vi "lab2_sim_modem.vi"() -> ()   [LabVIEW 2014]
uses:
  <vilib>/Addons/Modulation/Digital/General/MT Generate Bits (Galois, PN Order).vi
  <vilib>/Addons/Modulation/Analog/support/mod_Set Error Source.vi
  <vilib>/Addons/Modulation/Digital/Support/Common/Validators/mod_Generate Bits Validate.vi
  <vilib>/Addons/Modulation/Digital/Support/Common/Validators/mod_AWGN Validate.vi
  <vilib>/Addons/Modulation/Digital/Impairments/subVIs/mod_createSeeds.vi
  <vilib>/Addons/Modulation/Digital/Support/Common/Validators/mod_Validate Samples Per Symbol.vi
  <vilib>/Addons/Modulation/Analog/support/Validators/mod_Validate Complex Waveform.vi
  <vilib>/Addons/Modulation/Analog/support/Validators/mod_WFErrorHandler.vi
  <vilib>/Addons/Modulation/Digital/Support/Common/Validators/mod_Generate Filter Coefficients Validate.vi
  <vilib>/Addons/Modulation/Digital/General/subVIs/mod_Generate Filter Coefficients.vi
  <vilib>/Addons/Modulation/Digital/General/subVIs/mod_Generate Bits PN Sequence.vi
  <vilib>/Addons/Modulation/Digital/General/MT Apply Pulse Shaping Filter (Generic).vi
  <vilib>/Analysis/1siggen.llb/Gaussian White Noise (obs 90).vi
  <vilib>/Addons/Modulation/Digital/General/MT Apply Matched Filter (Generic).vi
  <vilib>/addons/Modulation/niDMT.lvlib
panel:
  out "ser/ber":dbl
  out "received symbols":u32
  out "error symbols":i32
  out "ser":dbl
  out "received bits":i32
  out "error bits":i32
  out "ber":dbl format="%#_5e"
  out "sync?":bool
  out "subarray":i16[](array[numeric])
  out "index map":u32[](array[numeric])
  out "output bit stream":i8[](array[numeric])
  in  "modulation":enum16{"PSK", "QAM"}(ring)
  in  "Gray code?":bool=TRUE
  out "size(s)":i32
  out "Received map":cdb[](graph)
  in  "Eb/N0 (10 dB)":dbl=10.0 format="%.2f"
  in  "samples per symbol":i32=16
  in  "filter parameter":dbl=0.5 format="%.2f"
  in  "filter length (symbols)":i32=8
  in  "pulse shaping filter (none)":T1(ring)=enum."Root Raised Cos"
  out "total bits":i32
  in  "total mod symbols":i32=2000 caption="total symbols"
  out "symbol map":cdb[](array[numeric])
  out "Transmitter map":cdb[](graph)
  in  "stop":bool
  in  "M-ARY":i32=4
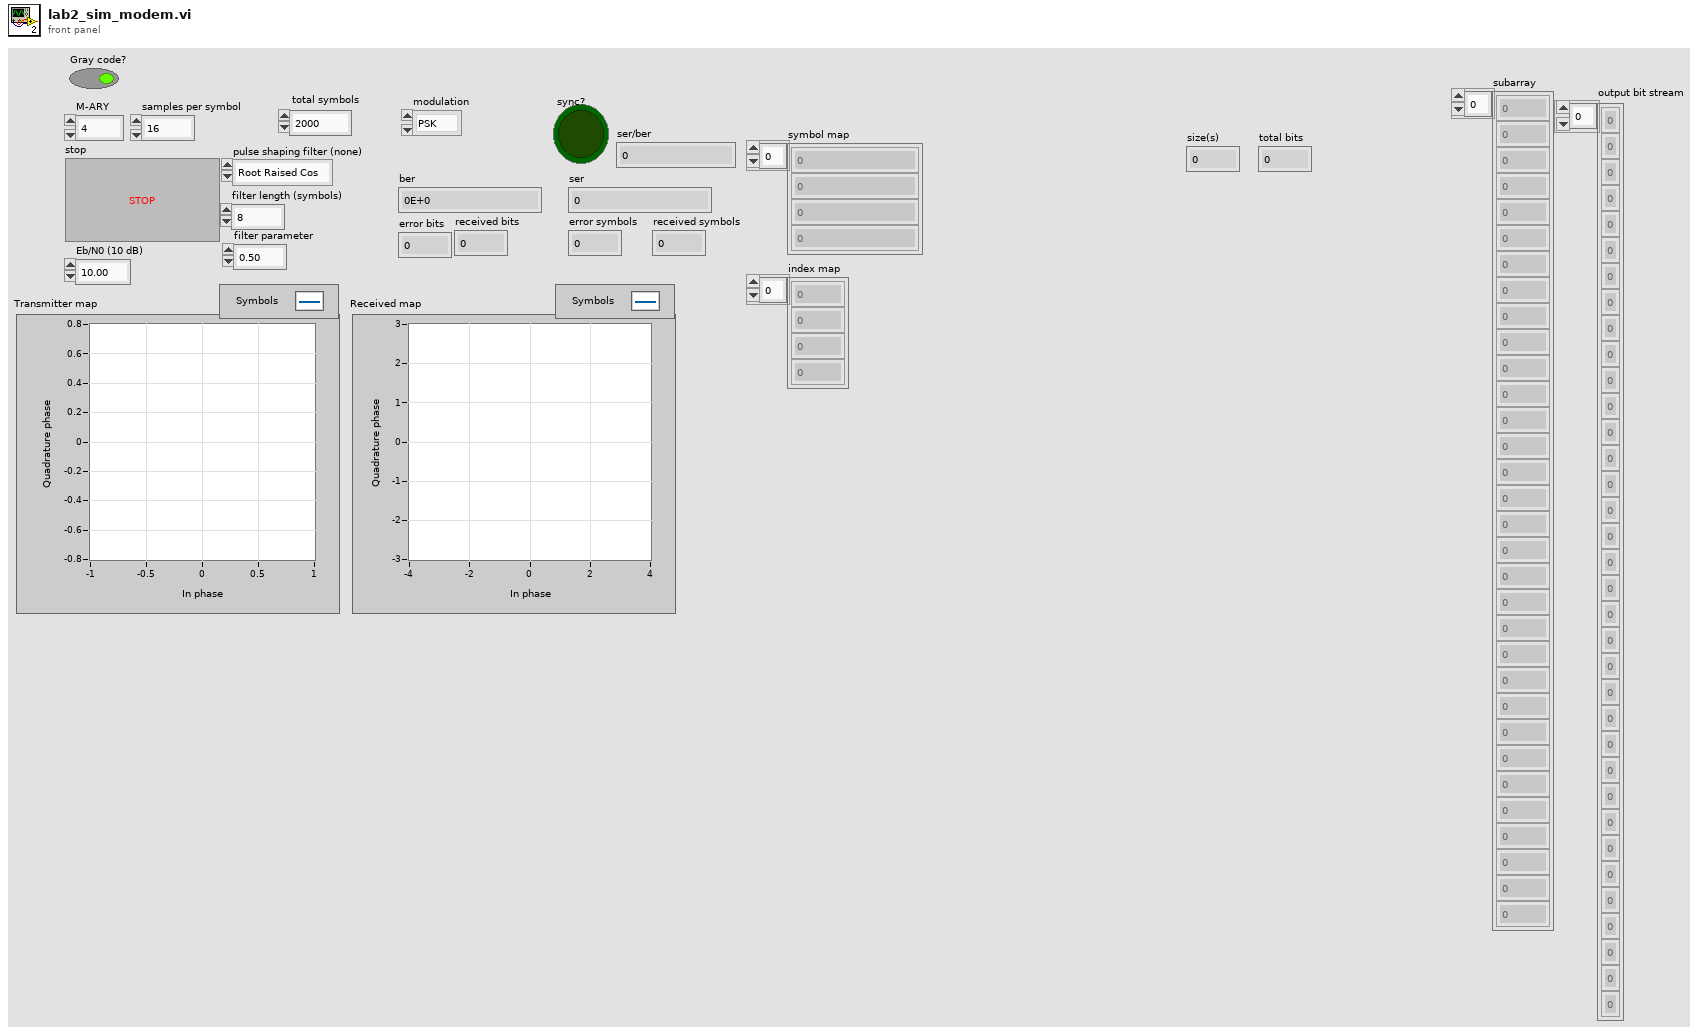
[diagram p1: front panel]
types:
  T1 = enum16{"none", "Raised Cosine", "Root Raised Cos", "Gaussian"}
  T2 = enum16{"FSK", "PSK", "QAM", "MSK", "PAM", "ASK", "CPM"}
  T3 = typedef "niAMT.lvlib/Complex Data Waveform.ctl" = cluster{"t0":dbl, "dt":dbl, "Y":cdb[]}
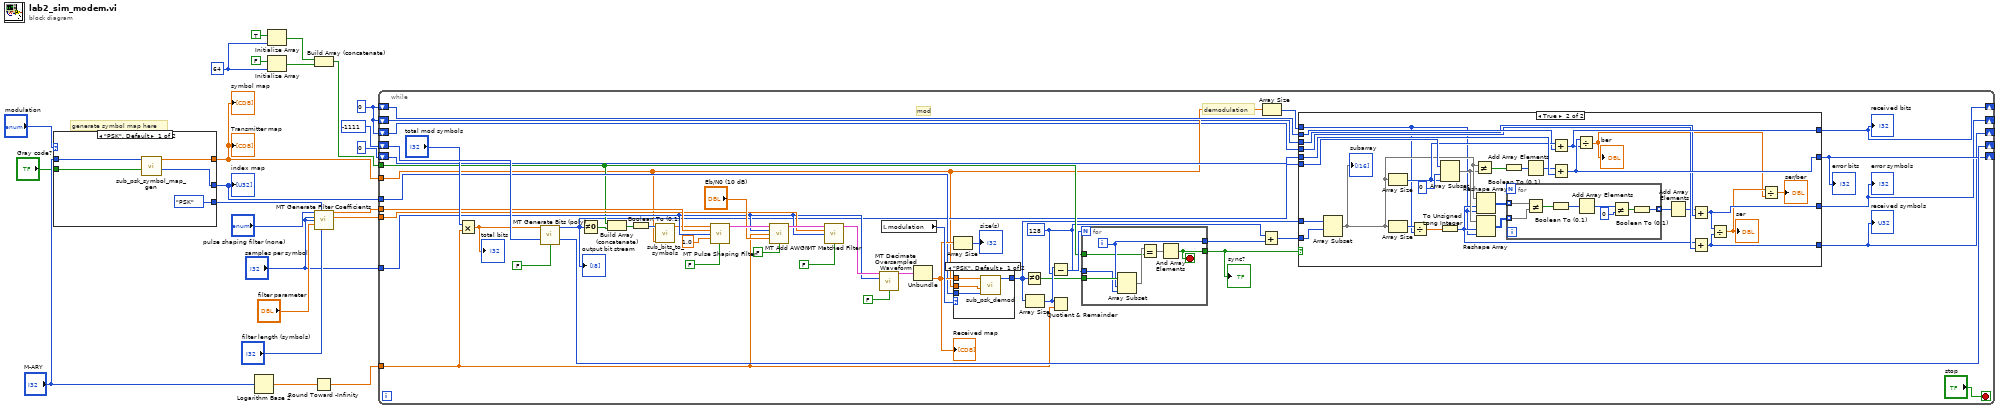
[diagram p0: block diagram]
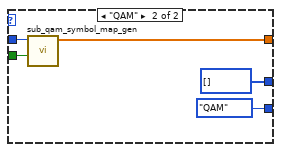
[diagram p2: hidden frame]
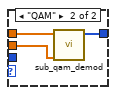
[diagram p4: hidden frame]
diagram:
  w1 = 0
  w3 = 64 ("dimension size")
  # "generate symbol map here"
  n1 = case shown="\"PSK\", Default" "modulation" {
    tunnel: "M-ARY" -> [w27 w33]
    tunnel: "Gray code?" -> [w28 w32]
    tunnel: [w26 w31] -> w11
    tunnel: [T2."PSK" ("modulation type") T2."QAM" ("modulation type")] -> w10
    tunnel: [w24 u32[] [] ("index map")] -> w9
    frame "PSK", Default {
      n2 = call "sub_psk_symbol_map_gen.vi"("Gray code?"=w28, "M-PSK"=w27) -> ("index map"=w24:u32[], "symbol map"=w26:cdb[])  [unwired: 8 in]
    }
    frame "QAM" {
      n3 = call "sub_qam_symbol_map_gen.vi"("Gray code?"=w32, "M-QAM"=w33) -> ("symbol map"=w31:cdb[])  [unwired: 9 in]
    }
  }
  "Transmitter map" <- w11
  "symbol map" <- w11
  "index map" <- w9
  n4 = Logarithm Base 2(1:"M-ARY") -> (0:w23:dbl)
  n5 = Initialize Array(TRUE, w3) -> (w8:bool[])
  n6 = Initialize Array(FALSE, w3) -> (w7:bool[])
  n7 = Round Toward -Infinity(1:w23) -> (0:w16:dbl)
  n8 = Build Array (concatenate)(w8, w7) -> (w4:bool[])
  n9 = call <vilib>:"MT Generate Filter Coefficients.vi"("pulse shaping filter (none)"="pulse shaping filter (none)", "modulation type"=w10, "pulse shaping samples per symbol (16)"="samples per symbol", "matched samples per symbol (16)"="samples per symbol", "filter parameter"="filter parameter", "filter length (symbols)"="filter length (symbols)") -> ("pulse shaping filter coefficients"=w18:dbl[], "matched filter coefficients"=w15:dbl[])  [unwired: 7 in, 1 out]
  n10 = while {
    tunnel: w11 -> [w39]
    shift-right: [w79] -> _
    shift-left: -1111 ("seed out") -> [w80]
    tunnel: w18 -> [w76]
    tunnel: "samples per symbol" -> [w66]
    tunnel: w16 -> [w60]
    tunnel: w15 -> [w68]
    tunnel: w9 -> [w61]
    tunnel: w4 -> [w55]
    shift-right: [w46] -> _
    shift-left: 0 -> [w47]
    shift-right: [w44] -> _
    shift-left: w1 -> [w45]
    shift-right: [w36] -> _
    shift-left: w1 -> [w38]
    shift-right: [w35] -> _
    shift-left: w1 -> [w37]
    stop <- "stop" stop-if-true
    w49 = 128
    # "demodulation"
    # "mod"
    n11 = Multiply(x="total mod symbols", y=w60) -> (x*y=w78:dbl)
    "total bits" <- w78
    n12 = call-poly <vilib>:"MT Generate Bits (poly).vi"("total bits (128)"=w78, "seed in (0xD6BF7DF2)"=w80, "reset? (T)"=FALSE) -> ("output bit stream"=w48:i8[], "seed out"=w79:i32)  [unwired: 10 in, 1 out]
    "output bit stream" <- w48
    n13 = Not Equal To 0?(x=w48) -> (x != 0?=w58:bool[])
    n14 = Build Array (concatenate)(w55, w58) -> (w42:bool[])
    n15 = Boolean To (0,1)(Boolean=w42) -> (0, 1=w41:i16[])
    n16 = call "sub_bits_to_symbols.vi"("symbol map"=w39, "bits"=w41) -> ("symbols"=w40:cdb[])  [unwired: 9 in]
    n17 = call-poly <vilib>:"MT Pulse Shaping Filter.vi"("symbols"=w40, "pulse shaping filter coefficients"=w76, "samples per symbol (16)"=w66, "symbol rate (Hz)"=1.0, "reset? (T)"=FALSE) -> ("output complex waveform"=w72:T3)  [unwired: 9 in, 1 out]
    n18 = call <vilib>:"MT Add AWGN.vi"("input complex waveform"=w72, "samples per symbol (16)"=w66, "bits per symbol (1)"=w60, "Eb/N0 (10 dB)"="Eb/N0 (10 dB)", "reset? (T)"=FALSE) -> ("output complex waveform"=w69:T3)  [unwired: 8 in, 2 out]
    n19 = call-poly <vilib>:"MT Matched Filter.vi"("input complex waveform"=w69, "matched filter coefficients"=w68, "samples per symbol (16)"=w66, "reset? (T)"=FALSE) -> ("output complex waveform"=w67:T3)  [unwired: 10 in, 1 out]
    n20 = call <vilib>:"MT Decimate Oversampled Waveform.vi"("input complex waveform"=w67, "decimation factor"=w66, "reset? (T)"=FALSE) -> ("output complex waveform"=w65:T3)  [unwired: 11 in, 1 out]
    n21 = local read "modulation"() -> (w63:enum16{"PSK", "QAM"})
    n22 = Unbundle(w65) -> ("Y"=w62:cdb[])  [unwired: 2 out]
    "Received map" <- w62
    n23 = Array Size(array=w62) -> (size(s)=→"size(s)":i32)
    n24 = case shown="\"PSK\", Default" w63 {
      tunnel: w62 -> [w133 w135]
      tunnel: w39 -> [w132 w136]
      tunnel: w61 -> [w131 _]
      tunnel: [w130 w134] -> w52
      frame "PSK", Default {
        n25 = call "sub_psk_demod.vi"("index map"=w131, "symbol map"=w132, "symbol"=w133) -> ("bitstream"=w130:i16[])  [unwired: 8 in]
      }
      frame "QAM" {
        n26 = call "sub_qam_demod.vi"("symbol map"=w136, "symbol"=w135) -> ("bitstream"=w134:i16[])  [unwired: 9 in]
      }
    }
    n27 = Not Equal To 0?(x=w52) -> (x != 0?=w53:bool[])
    n28 = Array Size(array=w52) -> (size(s)=w57:i32)
    n29 = Subtract(x=w57, y=w49) -> (x-y=w56:i32)
    n30 = Quotient & Remainder(x=w57, y=w60) -> ()  [unwired: 2 out]
    n31 = for {
      N: w56 -> [_]
      tunnel: w53 -> [w129]
      tunnel: [w128] -> w51
      tunnel: w49 -> [w127]
      tunnel: w55 -> [w125]
      tunnel: [w123] -> w54
      i -> [w128]
      stop <- w123 stop-if-true
      n32 = Array Subset(array=w129, index=w128, length=w127) -> (w126:bool[])
      n33 = Equal?(x=w126, y=w125) -> (x = y?=w124:bool[])
      n34 = And Array Elements(Boolean array=w124) -> (logical AND=w123:bool)
    }
    "sync?" <- w54
    n35 = Add(x=w49, y=w51) -> (x+y=w50:i32)
    n36 = Array Size(array=w39) -> (size(s)=w34:i32)
    n37 = case shown="True" w54 {
      tunnel: w52 -> [_ w114]
      tunnel: w50 -> [_ w113]
      tunnel: w48 -> [_ w111]
      tunnel: w47 -> [w85 w108]
      tunnel: [w85 w106] -> w46
      tunnel: w45 -> [w84 w104]
      tunnel: [w84 w103] -> w44
      tunnel: w38 -> [w83 w93]
      tunnel: w37 -> [w82 w95]
      tunnel: [w82 w91] -> w35
      tunnel: [w83 w90] -> w36
      tunnel: w34 -> [_ w89]
      frame False {
      }
      frame True {
        n38 = Array Subset(array=w114, index=w113) -> (w100:i16[])  [unwired: 1 in]
        "subarray" <- w100
        n39 = Array Size(array=w100) -> (size(s)=w105:i32)
        n40 = Array Size(array=w100) -> (size(s)=w102:i32)
        n41 = Divide(x=w102, y=w89) -> (x/y=w101:dbl)
        n42 = Array Subset(array=w111, index=0, length=w105) -> (w99:i8[])
        n43 = To Unsigned Long Integer(number=w101) -> (unsigned 32bit integer=w94:u32)
        n44 = Not Equal?(x=w100, y=w99) -> (x != y?=w110:bool[])
        n45 = Reshape Array(w100, w94, w89) -> (w98:i16[][])
        n46 = Reshape Array(w99, w94, w89) -> (w97:i8[][])
        n47 = Boolean To (0,1)(Boolean=w110) -> (0, 1=w109:i16[])
        n48 = for {
          tunnel: w98 -> [w122] mode=indexing
          tunnel: w97 -> [w121] mode=indexing
          tunnel: [w115] -> w96 mode=indexing
          n49 = Not Equal?(x=w122, y=w121) -> (x != y?=w120:bool[])
          n50 = Boolean To (0,1)(Boolean=w120) -> (0, 1=w119:i16[])
          n51 = Add Array Elements(numeric array=w119) -> (sum=w118:i16)
          n52 = Not Equal?(x=w118, y=0) -> (x != y?=w116:bool)
          n53 = Boolean To (0,1)(Boolean=w116) -> (0, 1=w115:i16)
        }
        n54 = Add Array Elements(numeric array=w109) -> (sum=w107:i16)
        n55 = Add(x=w105, y=w104) -> (x+y=w103:i32)
        n56 = Add(x=w107, y=w108) -> (x+y=w106:i32)
        n57 = Divide(x=w106, y=w103) -> (x/y=w87:dbl)
        "ber" <- w87
        n58 = Add Array Elements(numeric array=w96) -> (sum=w92:i16)
        n59 = Add(x=w92, y=w93) -> (x+y=w90:i32)
        n60 = Add(x=w94, y=w95) -> (x+y=w91:u32)
        n61 = Divide(x=w90, y=w91) -> (x/y=w88:dbl)
        "ser" <- w88
        n62 = Divide(x=w88, y=w87) -> (x/y=→"ser/ber":dbl)
      }
    }
    "error bits" <- w46
    "received bits" <- w44
    "error symbols" <- w36
    "received symbols" <- w35
  }
